vi "Swerve Wheel.vi"(2 "Wheel":T1(ring), 3 "Debug?":bool, 4 "Inputs":dbl[](array[numeric])) -> (0 "Speed":dbl)   [LabVIEW 2015]
uses:
  <vilib>/addons/control/pid/pid.llb/PID (DBL).vi
  <vilib>/addons/control/pid/NI_PID_pid.lvlib
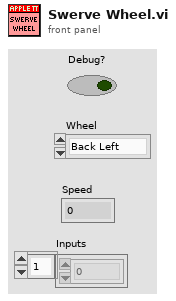
[diagram p1: front panel]
types:
  T1 = enum16{"Back Left", "Back Right", "Front Left", "Front Right"}
  T2 = enum16{"Z", "Y", "X", "Rot. Point X", "Rot. Point Y", "Width/2", "Max", "Length/2"}
  T3 = enum16{"Z Axis", "Y", "X", "Rot. Point X", "Rot. Point Y", "Width/2", "Max", "Length/2"}
  T4 = cluster{"proportional gain (Kc)":dbl, "integral time (Ti, min)":dbl, "derivative time (Td, min)":dbl}
  T5 = typedef "WPI_AnalogChannelDevRef.ctl" = cluster{"DevStatus":errorcluster, "Analog Channel":T6}
  T6 = typedef "FPGA_AIChannel.ctl" = enum8{"AI 0", "AI 1", "AI 2", "AI 3", "AI MXP 0", "AI MXP 1", "AI MXP 2", "AI MXP 3", "Invalid"}
  T7 = typedef "WPI_MotorControlDeviceRef.ctl" = cluster{"DeviceStatus":errorcluster, "Type":T8, "PWM":cluster{"PWM Channel":T9, "DeadBand":T10}, "CAN":cluster{"Device Number":u8, "Control Mode":T11, "Semaphore":T12, "Max Vout":dbl, "TalonSRX Control Mode":T13}, "Invert":bool}
  T8 = typedef "WPI_MotorControlType.ctl" = enum16{"PWM", "CAN", "CANTalonSRX"}
  T9 = typedef "FPGA_DIOPWMChannel.ctl" = enum8{"PWM 0", "PWM 1", "PWM 2", "PWM 3", "PWM 4", "PWM 5", "PWM 6", "PWM 7", "PWM 8", "PWM 9", "PWM MXP 0", "PWM MXP 1", "PWM MXP 2", "PWM MXP 3", "PWM MXP 4", "PWM MXP 5", "PWM MXP 6", "PWM MXP 7", "PWM MXP 8", "PWM MXP 9", "Invalid"}
  T10 = typedef "WPI_PWMDeadband.ctl" = cluster{"Name":string, "maxPositivePwm":i32, "minPositivePwm":i32, "centerPwm":i32, "maxNegativePwm":i32, "minNegativePwm":i32, "angularRange":u16}
  T11 = typedef "WPI_CANJaguar_ControlMode.ctl" = enum8{"Percent VBus", "Current", "Speed", "Position", "Voltage"}
  T12 = typedef "Semaphore RefNum" = refnum<k1>
  T13 = typedef "WPI_CANTalonSRX_APIControlMode.ctl" = enum8{"Percent VBus", "Speed", "Position", "Slave", "Unchanged / Invalid", "Voltage Compensation", "Current", "Motion Profile"}
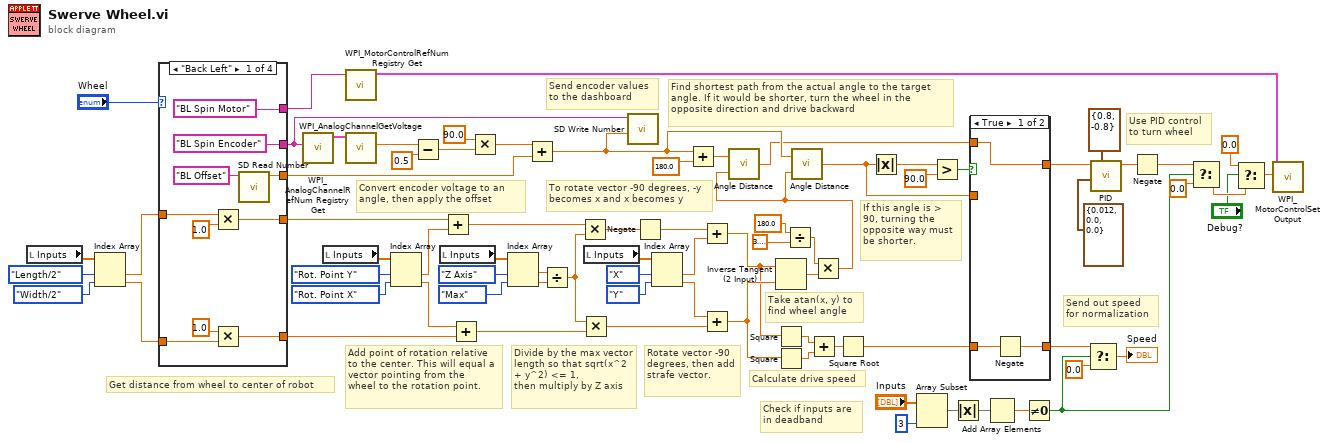
[diagram p0: block diagram]
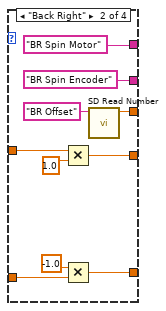
[diagram p3: hidden frame]
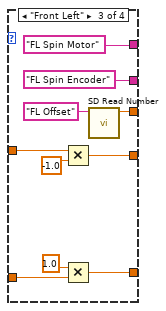
[diagram p4: hidden frame]
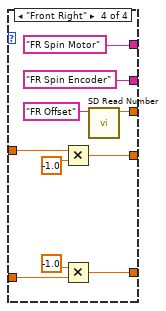
[diagram p5: hidden frame]
diagram:
  # "Send encoder values \nto the dashboard"
  # "To rotate vector -90 degrees, -y becomes x and x becomes y"
  # "Divide by the max vector length so that sqrt(x^2 + y^2) <= 1,\nthen multiply by Z axis"
  # "Add point of rotation relative to the center. This will equal a vector pointing from the\nwheel to the rotation point."
  # "Send out speed\nfor normalization"
  # "Check if inputs are\nin deadband"
  # "Convert encoder voltage to an angle, then apply the offset"
  # "If this angle is > 90, turning the opposite way must be shorter."
  # "Use PID control\nto turn wheel"
  # "Find shortest path from the actual angle to the target angle. If it would be shorter, turn the wheel in the opposite direction and drive backward"
  # "Take atan(x, y) to find wheel angle"
  # "Calculate drive speed"
  # "Rotate vector -90 degrees, then add strafe vector."
  # "Get distance from wheel to center of robot"
  n1 = local read "Inputs"() -> (w15:dbl[])
  n2 = Index Array(array=w15, index #1=T2."Length/2", index #2=T2."Width/2") -> (element #1=w13:dbl, element #2=w12:dbl)
  n3 = case shown="\"Back Left\"" "Wheel" {
    tunnel: ["BL Spin Encoder" "BR Spin Encoder" "FL Spin Encoder" "FR Spin Encoder"] -> w42
    tunnel: ["BL Spin Motor" "BR Spin Motor" "FL Spin Motor" "FR Spin Motor"] -> w62
    tunnel: [w84 w94 w104 w114] -> w52
    tunnel: w13 -> [w82 w92 w102 w112]
    tunnel: w12 -> [w80 w90 w100 w110]
    tunnel: [w79 w89 w99 w109] -> w39
    tunnel: [w78 w88 w98 w108] -> w35
    frame "Back Left" {
      n4 = Multiply(x=w82, y=1.0) -> (x*y=w79:dbl)
      n5 = Multiply(x=1.0 ("y"), y=w80) -> (x*y=w78:dbl)
      n6 = call <vilib>:"SD Read Number.vi"("Name"="BL Offset") -> ("Numeric"=w84:dbl)  [unwired: 8 in, 2 out]
    }
    frame "Back Right" {
      n7 = Multiply(x=w92, y=1.0) -> (x*y=w89:dbl)
      n8 = Multiply(x=-1.0 ("y"), y=w90) -> (x*y=w88:dbl)
      n9 = call <vilib>:"SD Read Number.vi"("Name"="BR Offset") -> ("Numeric"=w94:dbl)  [unwired: 8 in, 2 out]
    }
    frame "Front Left" {
      n10 = Multiply(x=w102, y=-1.0) -> (x*y=w99:dbl)
      n11 = Multiply(x=1.0 ("y"), y=w100) -> (x*y=w98:dbl)
      n12 = call <vilib>:"SD Read Number.vi"("Name"="FL Offset") -> ("Numeric"=w104:dbl)  [unwired: 8 in, 2 out]
    }
    frame "Front Right" {
      n13 = Multiply(x=w112, y=-1.0) -> (x*y=w109:dbl)
      n14 = Multiply(x=-1.0 ("y"), y=w110) -> (x*y=w108:dbl)
      n15 = call <vilib>:"SD Read Number.vi"("Name"="FR Offset") -> ("Numeric"=w114:dbl)  [unwired: 8 in, 2 out]
    }
  }
  n16 = call <vilib>:"WPI_AnalogChannelRefNum Registry Get.vi"("refnum name"=w42) -> ("AIDeviceRef"=w57:T5)  [unwired: 9 in, 1 out]
  n17 = local read "Inputs"() -> (w37:dbl[])
  n18 = call <vilib>:"WPI_MotorControlRefNum Registry Get.vi"("refnum name"=w62) -> ("MotorControlDevRef"=w75:T7)  [unwired: 9 in, 1 out]
  n19 = call <vilib>:"WPI_AnalogChannelGetVoltage.vi"("AIDeviceRef"=w57) -> ("Voltage"=w56:dbl)  [unwired: 8 in, 2 out]
  n20 = Index Array(array=w37, index #1=T2."Rot. Point Y", index #2=T2."Rot. Point X") -> (element #1=w33:dbl, element #2=w34:dbl)
  n21 = Subtract(x=w56, y=0.5) -> (x-y=w55:dbl)
  n22 = local read "Inputs"() -> (w31:dbl[])
  n23 = Add(x=w39, y=w33) -> (x+y=w8:dbl)
  n24 = Add(x=w34, y=w35) -> (x+y=w27:dbl)
  n25 = Multiply(x=90.0 ("y"), y=w55) -> (x*y=w53:dbl)
  n26 = Index Array(array=w31, index #1=T3."Z Axis", index #2=T2."Max") -> (element #1=w28:dbl, element #2=w29:dbl)
  n27 = Add(x=w53, y=w52) -> (x+y=w6:dbl)
  n28 = Divide(x=w28, y=w29) -> (x/y=w26:dbl)
  n29 = Multiply(x=w8, y=w26) -> (x*y=w10:dbl)
  n30 = Multiply(x=w26, y=w27) -> (x*y=w21:dbl)
  n31 = local read "Inputs"() -> (w24:dbl[])
  n32 = call <vilib>:"SD Write Number.vi"("Numeric"=w6, "Name"=w42) -> ()  [unwired: 8 in, 2 out]
  n33 = Negate(x=w10) -> (-x=w9:dbl)
  n34 = Index Array(array=w24, index #1=T2."X", index #2=T2."Y") -> (element #1=w19:dbl, element #2=w20:dbl)
  n35 = Add(x=w6, y=180.0 ("f")) -> (x+y=w49:dbl)
  n36 = Add(x=w9, y=w19) -> (x+y=w17:dbl)
  n37 = Add(x=w20, y=w21) -> (x+y=w18:dbl)
  n38 = Inverse Tangent (2 Input)(1:w18, 2:w17) -> (0:w73:dbl)
  n39 = Square(x=w17) -> (x^2=w22:dbl)
  n40 = Square(x=w18) -> (x^2=w72:dbl)
  n41 = Divide(x=180.0 ("y"), y=3.141592653589793) -> (x/y=w70:dbl)
  n42 = Add(x=w22, y=w72) -> (x+y=w71:dbl)
  n43 = Multiply(x=w70, y=w73) -> (x*y=w11:dbl)
  n44 = call "Angle Distance.vi"("target angle"=w11, "current angle"=w49) -> ("distance"=w5:dbl)
  n45 = call "Angle Distance.vi"("target angle"=w11, "current angle"=w6) -> ("distance"=w64:dbl)
  n46 = Square Root(x=w71) -> (sqrt(x)=w63:dbl)
  n47 = Absolute Value(x=w64) -> (abs(x)=w65:dbl)
  n48 = Array Subset(array="Inputs", length=3) -> (w48:dbl[])  [unwired: 1 in]
  n49 = Greater?(x=w65, y=90.0) -> (0:w44:bool)
  n50 = Absolute Value(x=w48) -> (abs(x)=w40:dbl[])
  n51 = case shown="True" w44 {
    tunnel: w5 -> [w118 _]
    tunnel: w64 -> [_ w122]
    tunnel: [w119 w121] -> w47
    tunnel: w63 -> [w120 w121]
    tunnel: [w118 w122] -> w59
    frame True {
      n52 = Negate(x=w120) -> (-x=w119:dbl)
    }
    frame False {
    }
  }
  n53 = Add Array Elements(numeric array=w40) -> (sum=w74:dbl)
  n54 = Not Equal To 0?(x=w74) -> (x != 0?=w43:bool)
  n55 = Select(t=w47, s=w43, f=0.0) -> (s? t:f=→"Speed":dbl)
  n56 = call-poly <vilib>:"PID.vi"("output range"=cluster{"output high":dbl, "output low":dbl} {"output high"=0.8, "output low"=-0.8}, "PID gains"=T4 {"proportional gain (Kc)"=0.012, "integral time (Ti, min)"=0.0, "derivative time (Td, min)"=0.0}, "setpoint"=w59) -> ("output"=w51:dbl)  [unwired: 7 in, 1 out]
  n57 = Negate(x=w51) -> (-x=w41:dbl)
  n58 = Select(t=w41, s=w43, f=0.0) -> (s? t:f=w3:dbl)
  n59 = Select(t=0.0, s="Debug?", f=w3) -> (s? t:f=w2:dbl)
  n60 = call <vilib>:"WPI_MotorControlSetOutput.vi"("Output"=w2, "MotorControlDevRef"=w75) -> ()  [unwired: 7 in, 3 out]
